vi "DataAcquisitionRamp.vi"(6 "stop":bool) -> (4 "lineIndex":u32)   [LabVIEW 2016]
uses:
  controls/Enum.ctl
  controls/FPGAVIreferenceTypeDef.ctl
  <vilib>/Utility/error.llb/Error Cluster From Error Code.vi
  <vilib>/rvi/errors/niLvFpgaAdjustHostInterfaceError.vi
  <vilib>/rvi/interface/common/niFpgaWaitOnOcc.vi
  <vilib>/rvi/interface/nirviReadWriteControl/nirviReadWriteControl.xnode
  FPGA Bitfiles/qnmController797_usbRIO_controllerFPGAmu_11012018-14h.lvbitx
  <vilib>/rvi/interface/nirviMethod/nirviMethod.xnode
  NiFpgaLv.dll
  <vilib>/FPGAPlugInAG/USB-7856R OEM/niLvFpga_ConfigureFifo_USB-7856R OEM.vi
  <vilib>/rvi/errors/niLvFpgaMergeErrorWithErrorCode.vi
panel:
  out "eltsRemaining":u32
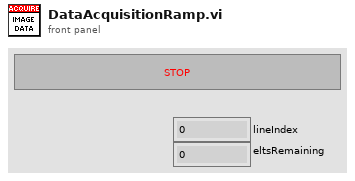
[diagram p1: front panel]
types:
  T1 = typedef "FPGAVIreferenceTypeDef.ctl" = refnum<k20>
  T2 = typedef "Enum.ctl" = enum16{"Init", "Read", "Write"}
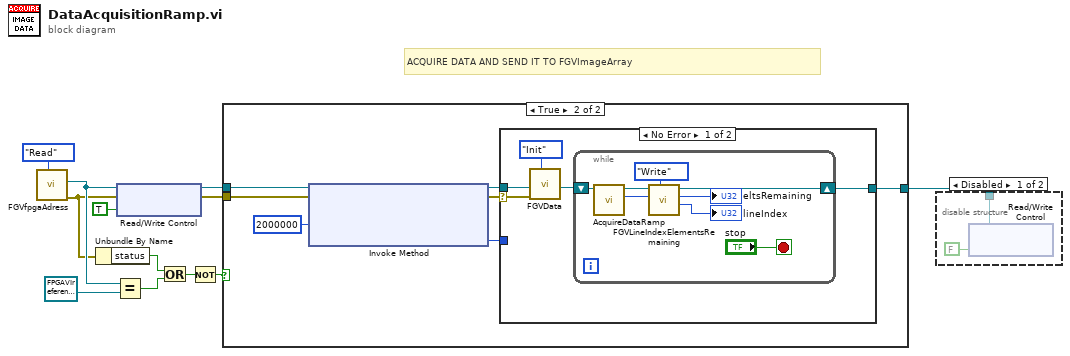
[diagram p0: block diagram]
diagram:
  # "ACQUIRE DATA AND SEND IT TO FGVImageArray"
  n1 = call "FGVfpgaAdress.vi"("Enum"=Enum."Read") -> ("error out"=w4:errorcluster, "FPGA VI Reference Out"=w5:T1)  [unwired: 6 in, 3 out]
  n2 = Unbundle By Name(w4) -> ("status"=w9:bool)
  n3 = Equal?(x=w5, y=T1 refnum ("FPGA VI Reference Out")) -> (x = y?=w8:bool)
  n4 = xnode "Read/Write Control"("FPGA VI Reference In"=w5, "error in"=w4, "hdt.o.enable"=TRUE) -> ("FPGA VI Reference Out"=w3:T1, "error out"=w2:errorcluster)
  n5 = Or(x=w9, y=w8) -> (x .or. y?=w10:bool)
  n6 = Not(x=w10) -> (.not. x?=w7:bool)
  n7 = case shown="True" w7 {
    tunnel: w3 -> [w13 w19]
    tunnel: w2 -> [_ w20]
    tunnel: [w13 w15] -> w6
    frame False {
    }
    frame True {
      n8 = xnode "Invoke Method"("FPGA VI Reference In"=w19, "error in"=w20, "Requested Depth"=u32 2000000) -> ("FPGA VI Reference Out"=w17:T1, "error out"=w16:errorcluster, "Actual Depth"=w14:u32)
      n9 = case shown="No Error" w16 {
        selector: w16 -> [w22 _]
        tunnel: w17 -> [w24 w32]
        tunnel: [w21 w32] -> w15
        tunnel: w14 -> [_ _]
        frame No Error {
          n10 = call "FGVData.vi"("Enum"=Enum."Init", "error in"=w22) -> ()  [unwired: 8 in, 2 out]
          n11 = while {
            shift-right: [w27] -> w21
            shift-left: w24 -> [w25]
            stop <- "stop" stop-if-true
            n12 = call "AcquireDataRamp.vi"("FPGA VI Reference In"=w25) -> ("Elements Remaining"=w30:u32, "FPGA VI Reference Out"=w27:T1)  [unwired: 8 in, 1 out]
            n13 = call "FGVLineIndexElementsRemaining.vi"("Enum"=Enum."Write", "elementsRemainingIn"=w30) -> ("lineIndexOut"=→"lineIndex":u32, "elementsRemainingOut"=→"eltsRemaining":u32)  [unwired: 6 in, 2 out]
          }
        }
        frame Error {
        }
      }
    }
  }
  n14 = disable-structure shown="Disabled" {
    disable-tunnel: w6 -> [w34 _]
    frame Disabled {
      n15 = xnode "Read/Write Control"("FPGA VI Reference In"=w34, "hdt.o.enable"=FALSE) -> ()  [unwired: 1 in, 2 out]
    }
    frame Enabled {
    }
  }
